vi "Generate.vi"(11 "Neopixel - FPGA In":refnum<class "Neopixel - FPGA.lvclass">) -> (2 "Digital Output":bool=TRUE, 3 "Neopixel - FPGA Out":refnum<class "Neopixel - FPGA.lvclass">)   [LabVIEW 2021, in "Neopixel - FPGA.lvclass"]
uses:
  Neopixel - FPGA.lvclass
  Private/Controls/Frame Pulse State.ctl
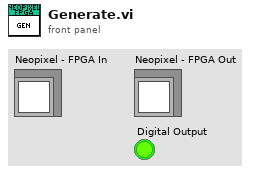
[diagram p1: front panel]
types:
  T1 = typedef "Neopixel - FPGA.lvclass/Frame Pulse State.ctl" = enum16{"Frame Pulse", "Delay"}
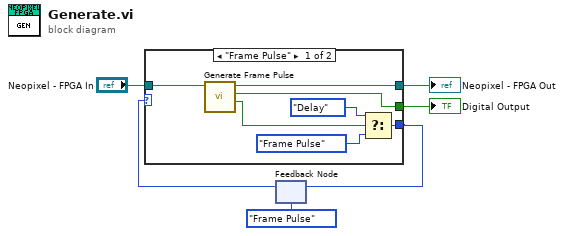
[diagram p0: block diagram]
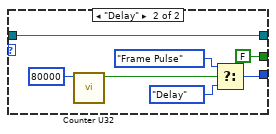
[diagram p2: hidden frame]
diagram:
  n1 = feedback #1(Frame_Pulse_State."Frame Pulse") -> (w2:T1)
  n2 = case shown="\"Frame Pulse\"" w2 {
    tunnel: "Neopixel - FPGA In" -> [w7 w20]
    tunnel: [w13 FALSE ("Pulse Output")] -> w5
    tunnel: [w12 w20] -> w4
    tunnel: [w8 w17] -> w3
    frame "Frame Pulse" {
      n3 = call "Generate Frame Pulse.vi"("Neopixel - FPGA In"=w7) -> ("Done"=w11:bool, "Pulse Output"=w13:bool, "Neopixel - FPGA Out"=w12:refnum<class "Neopixel - FPGA.lvclass">)  [unwired: 8 in]
      n4 = Select(t=Frame_Pulse_State."Delay", s=w11, f=Frame_Pulse_State."Frame Pulse") -> (s? t:f=w8:T1)
    }
    frame "Delay" {
      n5 = call "Counter U32.vi"("Count To"=u32 80000) -> ("Value Reached"=w14:bool)  [unwired: 9 in, 1 out]
      n6 = Select(t=Frame_Pulse_State."Frame Pulse", s=w14, f=Frame_Pulse_State."Delay") -> (s? t:f=w17:T1)
    }
  }
  "Neopixel - FPGA Out" <- w4
  "Digital Output" <- w5
  n7 = feedback-in #1(w3) -> ()
